vi "Same Buffers.vi"(8 "error in (no error)":errorcluster, 10 "Buffers 2":refnum<class "Buffers.lvclass">, 11 "Buffers 1":refnum<class "Buffers.lvclass">) -> (0 "error out":errorcluster, 2 "same buffers?":bool)   [LabVIEW 2017, in "DSF Core.lvlib" / "Buffers.lvclass"]
uses:
  Buffers.lvclass
  Buffer/Buffer.lvclass
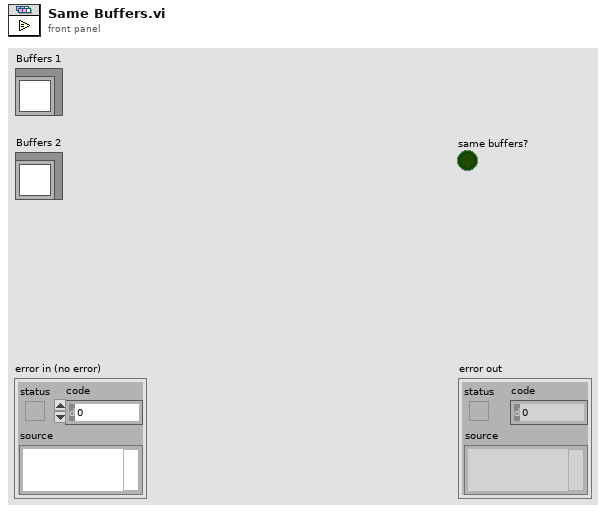
[diagram p1: front panel]
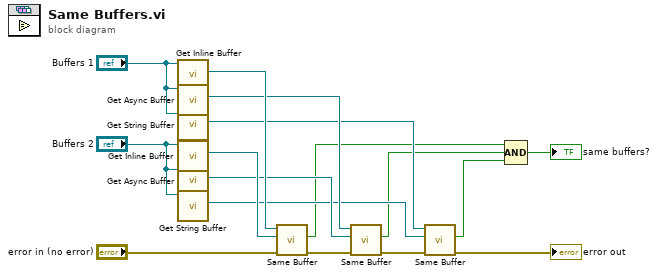
[diagram p0: block diagram]
diagram:
  n1 = call "Get Inline Buffer.vi"("Buffers in"="Buffers 1") -> ("Inline Buffer"=w14:refnum<class "Buffer.lvclass">)  [unwired: 9 in, 1 out]
  n2 = call "Get Async Buffer.vi"("Buffers in"="Buffers 1") -> ("Async Buffer"=w9:refnum<class "Buffer.lvclass">)  [unwired: 9 in, 1 out]
  n3 = call "Get String Buffer.vi"("Buffers in"="Buffers 1") -> ("String Buffer"=w7:refnum<class "Buffer.lvclass">)  [unwired: 9 in, 1 out]
  n4 = call "Get Inline Buffer.vi"("Buffers in"="Buffers 2") -> ("Inline Buffer"=w13:refnum<class "Buffer.lvclass">)  [unwired: 9 in, 1 out]
  n5 = call "Get Async Buffer.vi"("Buffers in"="Buffers 2") -> ("Async Buffer"=w8:refnum<class "Buffer.lvclass">)  [unwired: 9 in, 1 out]
  n6 = call "Get String Buffer.vi"("Buffers in"="Buffers 2") -> ("String Buffer"=w6:refnum<class "Buffer.lvclass">)  [unwired: 9 in, 1 out]
  n7 = call "Same Buffer.vi"("error in (no error)"="error in (no error)", "Buffer 2"=w13, "Buffer 1"=w14) -> ("error out"=w11:errorcluster, "same buffer?"=w3:bool)  [unwired: 7 in]
  n8 = call "Same Buffer.vi"("error in (no error)"=w11, "Buffer 2"=w8, "Buffer 1"=w9) -> ("error out"=w10:errorcluster, "same buffer?"=w4:bool)  [unwired: 7 in]
  n9 = call "Same Buffer.vi"("error in (no error)"=w10, "Buffer 2"=w6, "Buffer 1"=w7) -> ("error out"=→"error out":errorcluster, "same buffer?"=w5:bool)  [unwired: 7 in]
  n10 = Compound Arithmetic op=AND(w3, w4, w5) -> (→"same buffers?":bool)
